vi "UART Write Byte Array.vi"(8 "Error In":errorcluster, 9 "Data":u8[](array[numeric]), 10 "UART Channel (0)":u8, 11 "LINX Resource":T1) -> (0 "Error Out":errorcluster, 3 "LINX Resource":T1)   [LabVIEW 2014, in "LMH-LINX.lvlib"]
doc: "Transmit an unsigned byte array on the specified UART channel."
uses:
  <vilib>/MakerHub/LINX/LMH-LINX.lvlib
  <vilib>/MakerHub/LINX/Private/Type Defs/LINX Ref.ctl
  <vilib>/MakerHub/LINX/Private/Type Defs/Platform.ctl
  <vilib>/MakerHub/LINX/Private/Type Defs/Interface.ctl
  <vilib>/MakerHub/LINX/Private/Device/Type Defs/LINX Device Config.ctl
  <vilib>/MakerHub/LINX/Private/Device/Type Defs/TCP Config.ctl
  <vilib>/MakerHub/LINX/Private/Device/Type Defs/Channels.ctl
  <vilib>/MakerHub/LINX/Private/Type Defs/Peripheral.ctl
  <vilib>/MakerHub/LINX/Private/Utilties/Generate Error.vi
  <vilib>/MakerHub/LINX/Private/Device/Device.lvlib
  <vilib>/MakerHub/LINX/Private/Local IO/Local IO.lvlib
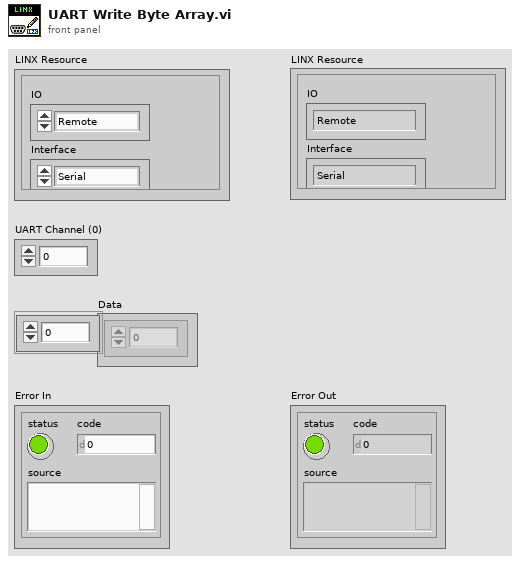
[diagram p1: front panel]
types:
  T1 = typedef "LMH-LINX.lvlib/LINX Ref.ctl" = cluster{"IO":T2, "Interface":T3, "LINX Device Config":T4}
  T2 = typedef "LMH-LINX.lvlib/Platform.ctl" = enum16{"Remote", "Local"}
  T3 = typedef "LMH-LINX.lvlib/Interface.ctl" = enum16{"Serial", "TCP"}
  T4 = typedef "LMH-LINX.lvlib/Device.lvlib/LINX Device Config.ctl" = cluster{"Interface":T3, "COM Port":refnum<visa-resource-name>, "TCP Configuration":T5, "Device Family":u8, "Device ID":u8, "Device Name":string, "TCP Ref":refnum<k5>, "Channels":T6}
  T5 = typedef "LMH-LINX.lvlib/Device.lvlib/TCP Config.ctl" = cluster{"IP Address":string, "Port":u16}
  T6 = typedef "LMH-LINX.lvlib/Channels.ctl" = cluster{"DI":u8[], "DO":u8[], "AI":u8[], "AO":u8[], "PWM":u8[], "QE":u8[], "UART":u8[], "I2C 2":u8[], "SPI":u8[], "CAN":u8[], "Servo":u8[], "AI Ref (V)":dbl, "AI Resolution (Bits)":u8, "AO Ref (V)":dbl, "AO Resolution (Bits)":u8}
  T7 = typedef "LMH-LINX.lvlib/Peripheral.ctl" = enum8{"DI", "DO", "AI", "AO", "PWM", "QE", "UART", "I2C", "SPI", "CAN", "Servo"}
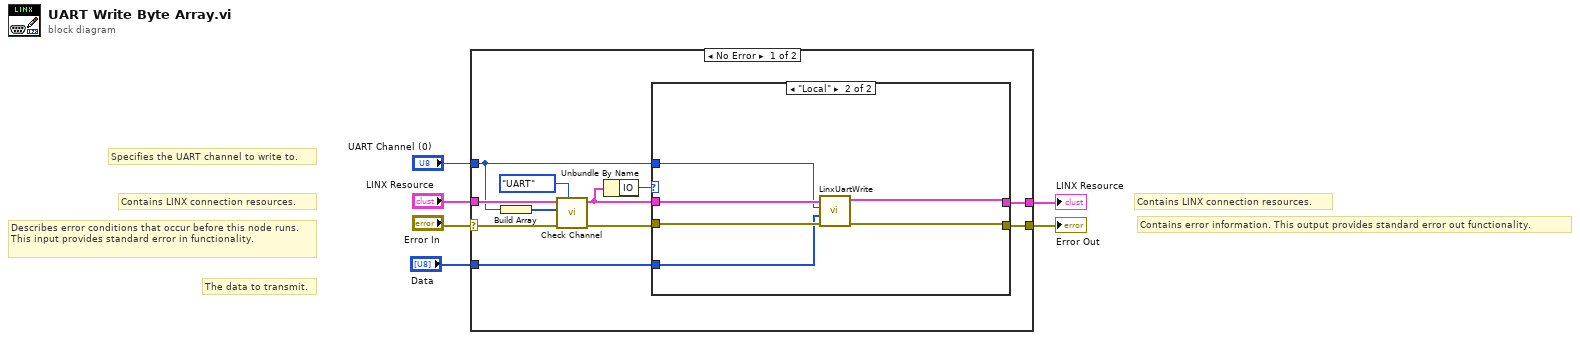
[diagram p0: block diagram]
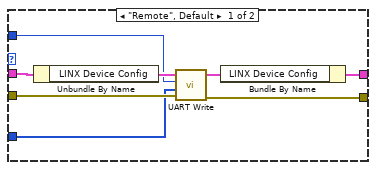
[diagram p2: hidden frame]
diagram:
  # "The data to transmit."
  # "Specifies the UART channel to write to."
  # "Contains LINX connection resources."
  # "Contains error information. This output provides standard error out functionality."
  # "Contains LINX connection resources."
  # "Describes error conditions that occur before this node runs. This input provides standard error in functionality."
  n1 = case shown="No Error" "Error In" {
    selector: "Error In" -> [w7 w33]
    tunnel: [w16 w33] -> w6
    tunnel: [w15 w32] -> w5
    tunnel: "LINX Resource" -> [w14 w32]
    tunnel: "UART Channel (0)" -> [w10 _]
    tunnel: "Data" -> [w8 _]
    frame No Error {
      n2 = Build Array(w10) -> (w11:u8[])
      n3 = call <vilib>:"Check Channel.vi"("Peripheral"=Peripheral."UART", "Error In"=w7, "Channels"=w11, "LINX Resource"=w14) -> ("Error Out"=w12:errorcluster, "LINX Resource"=w13:T1)  [unwired: 5 in, 1 out]
      n4 = Unbundle By Name(w13) -> ("IO"=w17:T2)
      n5 = case shown="\"Local\"" w17 {
        tunnel: w12 -> [w22 w31]
        tunnel: w13 -> [w25 w28]
        tunnel: [w23 w30] -> w16
        tunnel: [w24 w29] -> w15
        tunnel: w10 -> [w19 w27]
        tunnel: w8 -> [w18 w26]
        frame "Remote", Default {
          n6 = Unbundle By Name(w25) -> ("LINX Device Config"=w21:T4)
          n7 = call <vilib>:"UART Write.vi"("Error In"=w22, "Data"=w18, "UART Channel"=w19, "LINX Device Config"=w21) -> ("Error Out"=w23:errorcluster, "LINX Device Config"=w20:T4)  [unwired: 6 in]
          n8 = Bundle By Name(cluster=w25, "LINX Device Config"=w20) -> (w24:T1)
        }
        frame "Local" {
          n9 = call <vilib>:"LinxUartWrite.vi"("Error In"=w31, "Data"=w26, "Uart Channel"=w27, "LINX Resource"=w28) -> ("Error Out"=w30:errorcluster, "LINX Resource"=w29:T1)  [unwired: 6 in]
        }
      }
    }
    frame Error {
    }
  }
  "Error Out" <- w6
  "LINX Resource" <- w5
